vi "subSave_AcquireCameraInfomation.vi"(0 "Camera in use":T2={"Model"="-", "Camera ID"="-", "Bits"=0}, 1 "Scale Info":T1, 2 "ROI":T3={"Bin"=1, "ROI"={"x offset"=0, "y offset"=0, "x width"=2048, "y width"=2048}} {"ROI"."x offset" min=1 max=512 step=1; "ROI"."y offset" min=1 max=512 step=1; "ROI"."x width" min=1 max=512 step=1; "ROI"."y width" min=1 max=512 step=1; "Bin" items=["1x1"=1, "2x2"=2, "4x4"=4]}, 3 "Exposure (msec)":dbl=100.0 min=1.0 max=5000.0 step=1.0) -> (5 "Text Out":string)   [LabVIEW 2015]
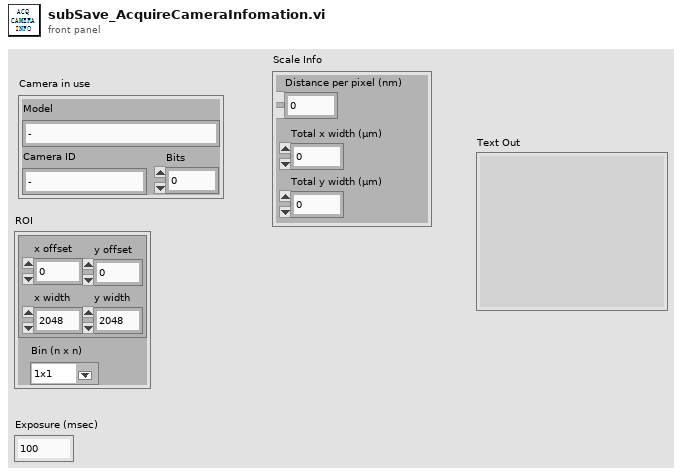
[diagram p1: front panel]
types:
  T1 = cluster{"Distance per pixel (nm)":dbl, "Total x width (μm)":dbl, "Total y width (μm)":dbl}
  T2 = cluster{"Model":string, "Camera ID":string, "Bits":i32}
  T3 = cluster{"Bin":u16, "ROI":cluster{"x offset":i32, "y offset":i32, "x width":i32, "y width":i32}}
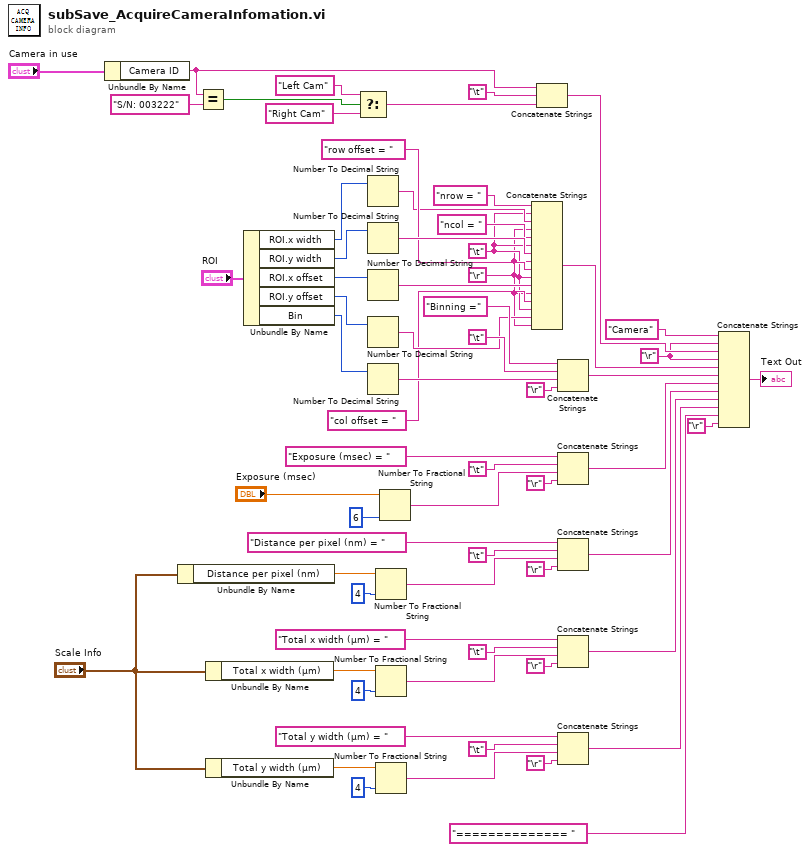
[diagram p0: block diagram]
diagram:
  w26 = "\r"
  w31 = "\r"
  w39 = "\t"
  n1 = Unbundle By Name("Camera in use") -> ("Camera ID"=w36:string)
  n2 = Unbundle By Name("Scale Info") -> ("Distance per pixel (nm)"=w19:dbl)
  n3 = Equal?(x=w36, y="S/N: 003222") -> (x = y?=w34:bool)
  n4 = Unbundle By Name("Scale Info") -> ("Total x width (μm)"=w6:dbl)
  n5 = Unbundle By Name("Scale Info") -> ("Total y width (μm)"=w5:dbl)
  n6 = Unbundle By Name("ROI") -> ("ROI.x width"=w41:i32, "ROI.y width"=w44:i32, "ROI.x offset"=w46:i32, "ROI.y offset"=w47:i32, "Bin"=w58:u16)
  n7 = Select(t="Left Cam" ("y"), s=w34, f="Right Cam" ("y")) -> (s? t:f=w30:string)
  n8 = Number To Decimal String(number=w41) -> (decimal integer string=w43:string)  [unwired: 1 in]
  n9 = Number To Decimal String(number=w44) -> (decimal integer string=w49:string)  [unwired: 1 in]
  n10 = Number To Decimal String(number=w46) -> (decimal integer string=w50:string)  [unwired: 1 in]
  n11 = Number To Decimal String(number=w47) -> (decimal integer string=w52:string)  [unwired: 1 in]
  n12 = Number To Decimal String(number=w58) -> (decimal integer string=w55:string)  [unwired: 1 in]
  n13 = Number To Fractional String(number=w19, precision (6)=i16 4) -> (F-format string=w24:string)  [unwired: 2 in]
  n14 = Number To Fractional String(number=w6, precision (6)=i16 4) -> (F-format string=w15:string)  [unwired: 2 in]
  n15 = Number To Fractional String(number=w5, precision (6)=i16 4) -> (F-format string=w11:string)  [unwired: 2 in]
  n16 = Number To Fractional String(number="Exposure (msec)", precision (6)=i16 6) -> (F-format string=w3:string)  [unwired: 2 in]
  n17 = Concatenate Strings("nrow = " ("string"), w39, w43, w31, "ncol = " ("string"), w39, w49, w31, "row offset = " ("string"), w39, w50, w31, "col offset = " ("string"), w39, w52, w31) -> (w37:string)
  n18 = Concatenate Strings(w36, "\t", w30) -> (w28:string)
  n19 = Concatenate Strings("Binning =", "\t", w55, "\r") -> (w62:string)
  n20 = Concatenate Strings("Exposure (msec) = " ("string"), "\t", w3, "\r") -> (w63:string)
  n21 = Concatenate Strings("Distance per pixel (nm) = " ("string"), "\t", w24, "\r") -> (w20:string)
  n22 = Concatenate Strings("Total x width (μm) = " ("string"), "\t", w15, "\r") -> (w13:string)
  n23 = Concatenate Strings("Total y width (μm) = " ("string"), "\t", w11, "\r") -> (w7:string)
  n24 = Concatenate Strings("Camera" ("string"), w26, w28, w26, w37, w62, w63, w20, w13, w7, "============== " ("string"), "\r") -> (→"Text Out":string)
